vi "Find External Path Combinations.vi"(11 "Found Common Paths in":string[](array[string])) -> (3 "External Path Combinations":string[](array[string]))   [LabVIEW 2019, in "Project.Dependencies Finder.lvlib"]
doc: "Find valid folder names and combinations of up to two names from given paths."
uses:
  Project.Dependencies Finder.lvlib
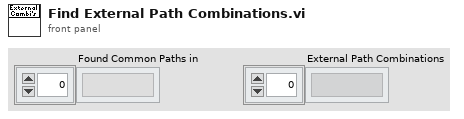
[diagram p1: front panel]
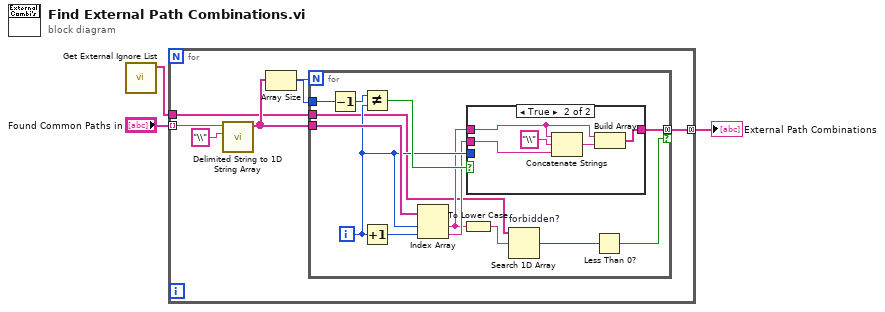
[diagram p0: block diagram]
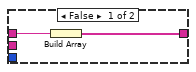
[diagram p2: hidden frame]
diagram:
  n1 = call "Get External Ignore List.vi"() -> ("Lower case external ignores"=w1:string[])  [unwired: 10 in, 1 out]
  n2 = for {
    tunnel: "Found Common Paths in" -> [w8] mode=indexing
    tunnel: [w5] -> w2 mode=concatenating
    tunnel: w1 -> [w4]
    n3 = call <vilib>:"Delimited String to 1D String Array.vi"("delimiter"="\\" ("search string"), "delimited string"=w8) -> ("string array"=w7:string[])  [unwired: 9 in]
    n4 = Array Size(array=w7) -> (size(s)=w6:i32)
    n5 = for {
      N: w6 -> [_]
      tunnel: w7 -> [w18]
      tunnel: w6 -> [w22]
      tunnel: [w19] -> w5 mode=concatenating if=w11
      tunnel: w4 -> [w10]
      i -> [w17]
      n6 = Decrement(x=w22) -> (x-1=w21:i32)
      n7 = Not Equal?(x=w21, y=w17) -> (x != y?=w20:bool)
      n8 = Increment(x=w17) -> (x+1=w16:i32)
      n9 = Index Array(array=w18, index #1=w17, index #2=w16) -> (element #1=w14:string, element #2=w15:string)
      n10 = To Lower Case(string=w14) -> (all lower case string=w13:string)
      n11 = case shown="True" w20 {
        tunnel: w17 -> [_ _]
        tunnel: [w24 w27] -> w19
        tunnel: w14 -> [w23 w26]
        tunnel: w15 -> [_ w25]
        frame False {
          n12 = Build Array(w23) -> (w24:string[])
        }
        frame True {
          n13 = Concatenate Strings(w26, "\\" ("search string"), w25) -> (w28:string)
          n14 = Build Array(w26, w28) -> (w27:string[])
        }
      }
      n15 = Search 1D Array "forbidden?"(1D array=w10, element=w13) -> (index of element=w12:i32)  [unwired: 1 in]
      n16 = Less Than 0?(x=w12) -> (x < 0?=w11:bool)
    }
  }
  "External Path Combinations" <- w2
